vi "Send Stop Event.vi"(8 "Error In":errorcluster, 11 "Display Panel V3 in":refnum<class "Display Panel V3.lvclass">) -> (0 "Error Out":errorcluster, 3 "Display Panel V3 out":refnum<class "Display Panel V3.lvclass">)   [LabVIEW 2013, in "Display Panel.lvlib" / "Display Panel V3.lvclass"]
uses:
  Display Panel V3.lvclass
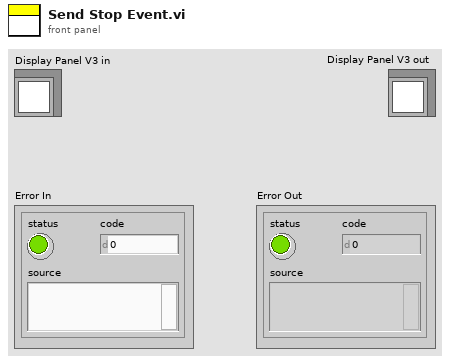
[diagram p1: front panel]
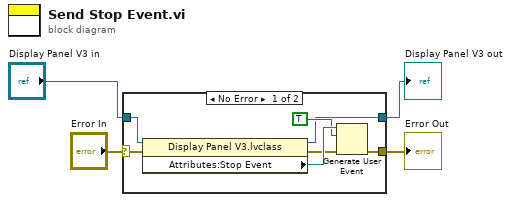
[diagram p0: block diagram]
diagram:
  n1 = case shown="No Error" "Error In" {
    selector: "Error In" -> [w8 w12]
    tunnel: "Display Panel V3 in" -> [w11 w13]
    tunnel: [w6 w12] -> w2
    tunnel: [w5 w13] -> w1
    frame No Error {
      n2 = property class="Display Panel V3.lvclass"(reference=w11, error in=w8) -> (reference out=w5:refnum<class "Display Panel V3.lvclass">, error out=w7:errorcluster, "Attributes:Stop Event"=w10:refnum<user-event>)
      n3 = Generate User Event(user event=w10, event data cluster=TRUE ("event data"), error in=w7) -> (error out=w6:errorcluster)  [unwired: 1 in, 1 out]
    }
    frame Error {
    }
  }
  "Display Panel V3 out" <- w1
  "Error Out" <- w2
